vi "serial_AUCT_p4.vi"() -> ()   [LabVIEW 2018]
uses:
  Controls created/Control 3.ctl
  Controls created/Control 4.ctl
  <vilib>/Instr/_visa.llb/VISA Configure Serial Port (Instr).vi
  <instrlib>/LeCroy Wave Series/Public/Data/Read Single Waveform.vi
  <vilib>/Utility/file.llb/Write Delimited Spreadsheet (DBL).vi
  <instrlib>/Siglent SDG X Series/Siglent SDG X Series.lvlib
  <instrlib>/LeCroy Wave Series/LeCroy Wave Series.lvlib
panel:
  in  "Tab Control":enum32{"Page 1", "Page 2", "Page 3"}(tab)
  in  "VISA resource":refnum<visa-resource-name>="COM5"
  in  "NR":i16=10
  in  "Set Speed (Steps/s)":i16=900 min=0 max=3000 step=50
  in  "Baud Rate":u32=9600
  out "Iteration #":i32
  in  "NT":i16=10
  out "Error":errorcluster
  in  "Arbitray Movement":bool
  out "stop motion":bool
  in  "MOTION":bool
  in  "?":i8(slide) step=2 scale=0.0..2.0
  in  "OK Button":bool
  out "# NT":i32
  in  "Scanning Distance(in mm)":i32=26
  in  "ms to wait(Translation)":u32=100
  out "Dis_step":dbl
  in  "milliseconds to wait":u32=100
  in  "ms to wait(Rotation)":u32=100
  in  "Directory":string="E:\\Ankur\\Labview\\Automation\\Data"
  out "Code Part Time":dbl[](array[numeric])
  in  "VISA Refnum in":refnum<visa-resource-name>="USB0::0xF4EC::0xEE38::SDG2XCAD2R3765::INSTR"
  in  "Channel (1:Channel 1)":i32(ring)=1 items=["Channel 1"=1, "Channel 2"=2]
  in  "Enable Output (T: Enable)":bool=TRUE
  in  "Amplitude (1.0 Vpp)":dbl=20.0 format="%#.3f"
  in  "Frequency (1000 Hz)":T1=1500000.0 format="%#.6g"
  in  "DC Offset (0.00 V) in":dbl
  in  "Waveform Function (0: Sine) in":u16(ring) items=["Sine", "Square", "Ramp", "DC", "Pulse", "Arb"]
  in  "Phase (0.0 degrees)":dbl=0.002 min=-360.0 max=360.0 format="%#.1g"
  in  "Fall (20 ns)":dbl=8.4e-09 format="%#.3g"
  in  "Duty (20%)":dbl=4.32 min=0.0001 max=100.0 format="%.4g"
  in  "Delay (0.00 s)":dbl min=-1000000.0 max=1000000.0
  in  "Rise (20 ns)":dbl=1.04e-08 format="%#.3g"
  in  "True To \ngenerate\n pulse":T2=TRUE
  out "VISA resource name out":refnum<visa-resource-name>
  out "error out":errorcluster
  out "Output Filename":path
  out "error out 2":errorcluster
  in  "format string":string="Channel: %g \nWavetype: %g \nAMP: %gV\nFreq: %gHz \nRiseTime: %gs \nFallTime: %gs \nDutyCycle: %g"
  out "Output Directory":path
  in  "File Directory":path=path "E:/Ankur/Labview/Automation/Data/Exp1"
  in  "Filename 2":string="wave_data"
  out "Oscilloscope\n Runnning":bool
  in  "stop":bool
  out "Waveform Data":waveform(dbl)(graph)
  in  "Source (0: Channel 1)":u16(ring) items=["Channel 1", "Channel 2", "Channel 3", "Channel 4", "Memory 1", "Memory 2", "Memory 3", "Memory 4", "Function 1", "Function 2", "Function 3", "Function 4", "Function 5", "Function 6", "Function 7", "Function 8"]
  in  "Perform Auto Setup?":bool
  in  "Save Files in Directory (In Oscilloscope)":string="D:\\Automation\\Data"
  in  "Filename":string="Title"
  in  "Path to save DATA":path=path "E:/Ankur/Labview/Automation/Files/Oscdata"
  out "Saved filename":string
  in  "Save File locally":bool
  out "Error Dsocom":errorcluster
  in  "VISA resource name":refnum<visa-resource-name>="LecroyHDO4024-1"
  in  "Reset Scope?":bool
  out "VISA DSO":refnum<visa-resource-name>
  # "For Rotational motion"
  # "For Translational Motion"
  # "For Translational motion"
  # "OFF"
  # "ON"
  # "Instr conn"
  # "Scan. loop"
  # "All Comb"
  # "Yes"
  # "No"
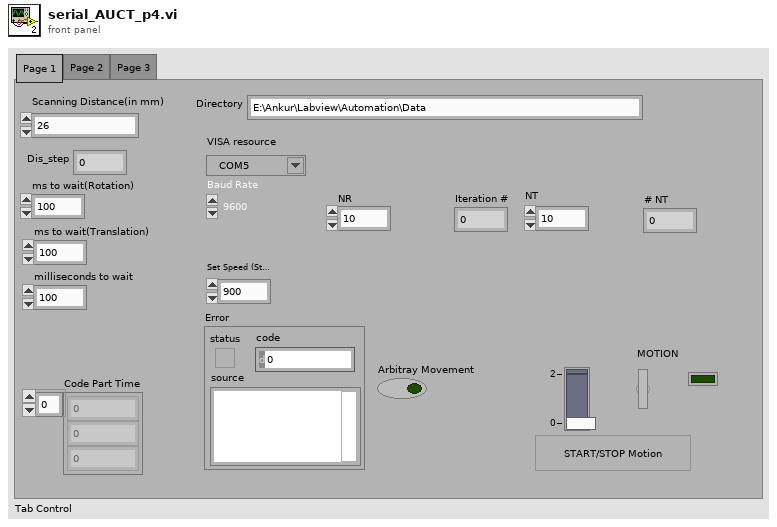
[diagram p1: front panel]
types:
  T1 = typedef "Control 3.ctl" = dbl
  T2 = typedef "Control 4.ctl" = bool
  T3 = enum16{"open", "replace", "create", "open or create", "replace or create", "replace or create with confirmation"}
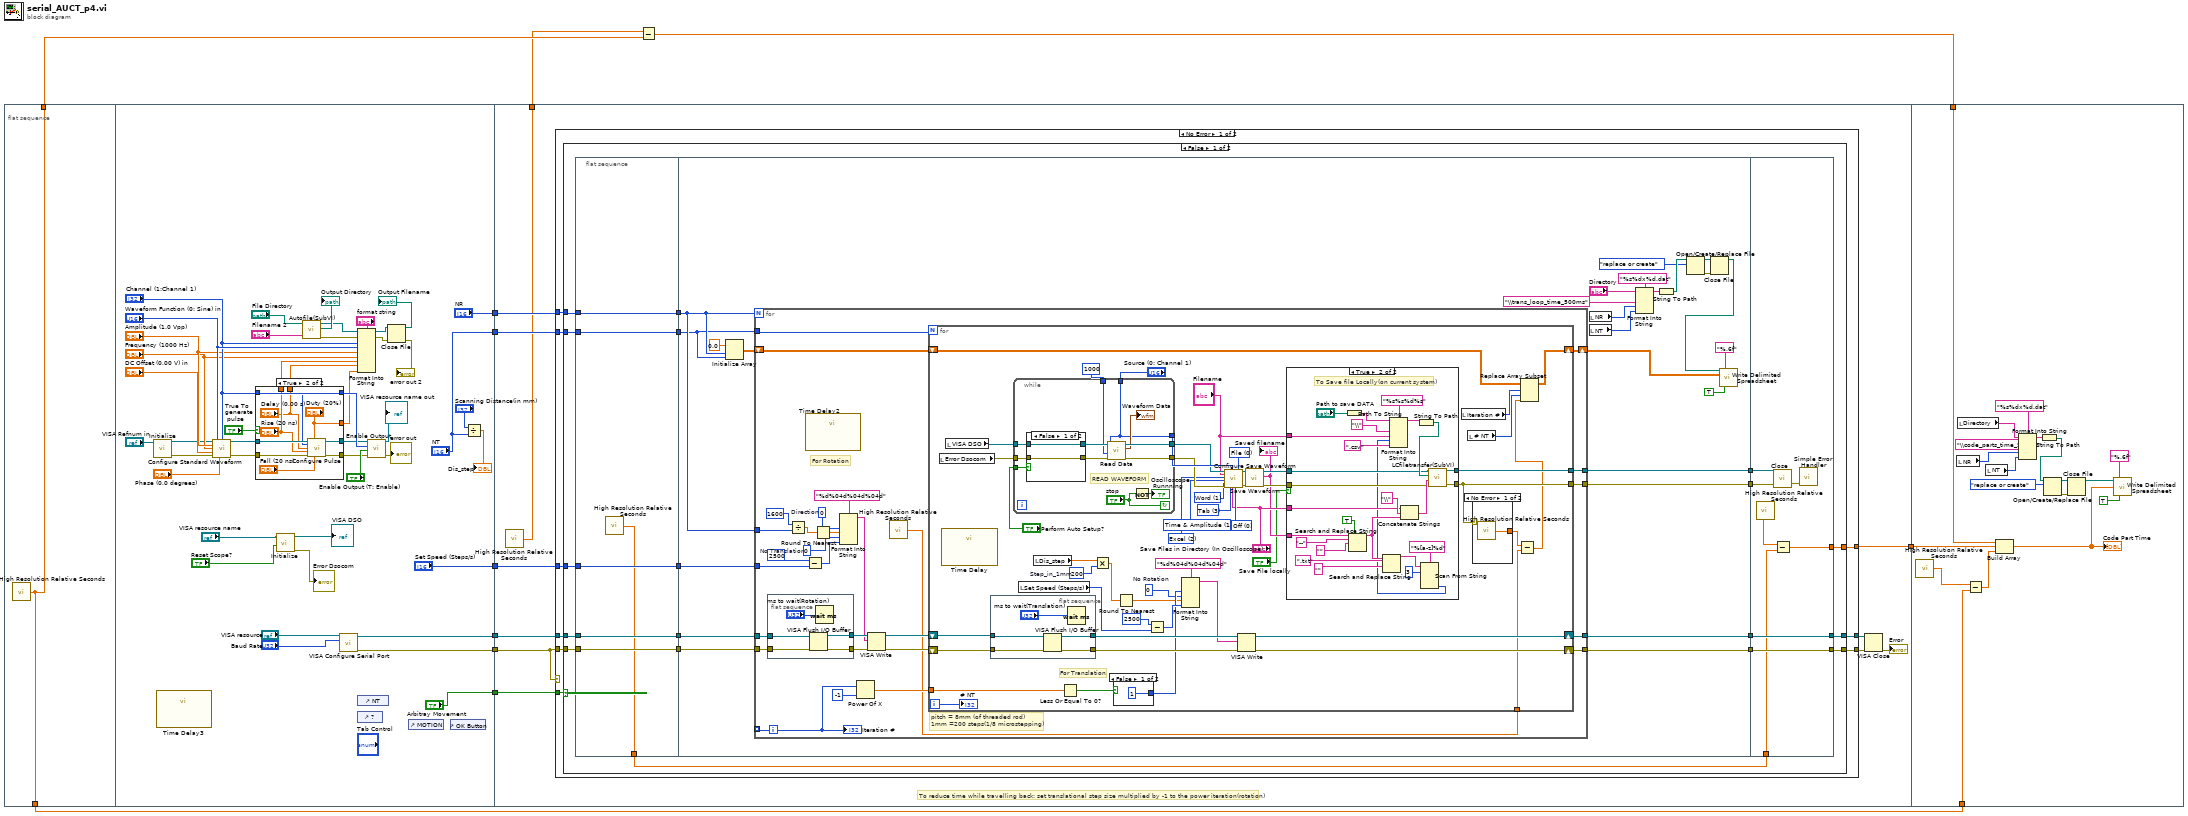
[diagram p0: block diagram]
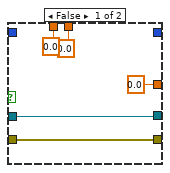
[diagram p2: hidden frame]
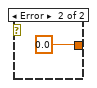
[diagram p3: hidden frame]
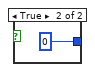
[diagram p4: hidden frame]
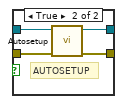
[diagram p6: hidden frame]
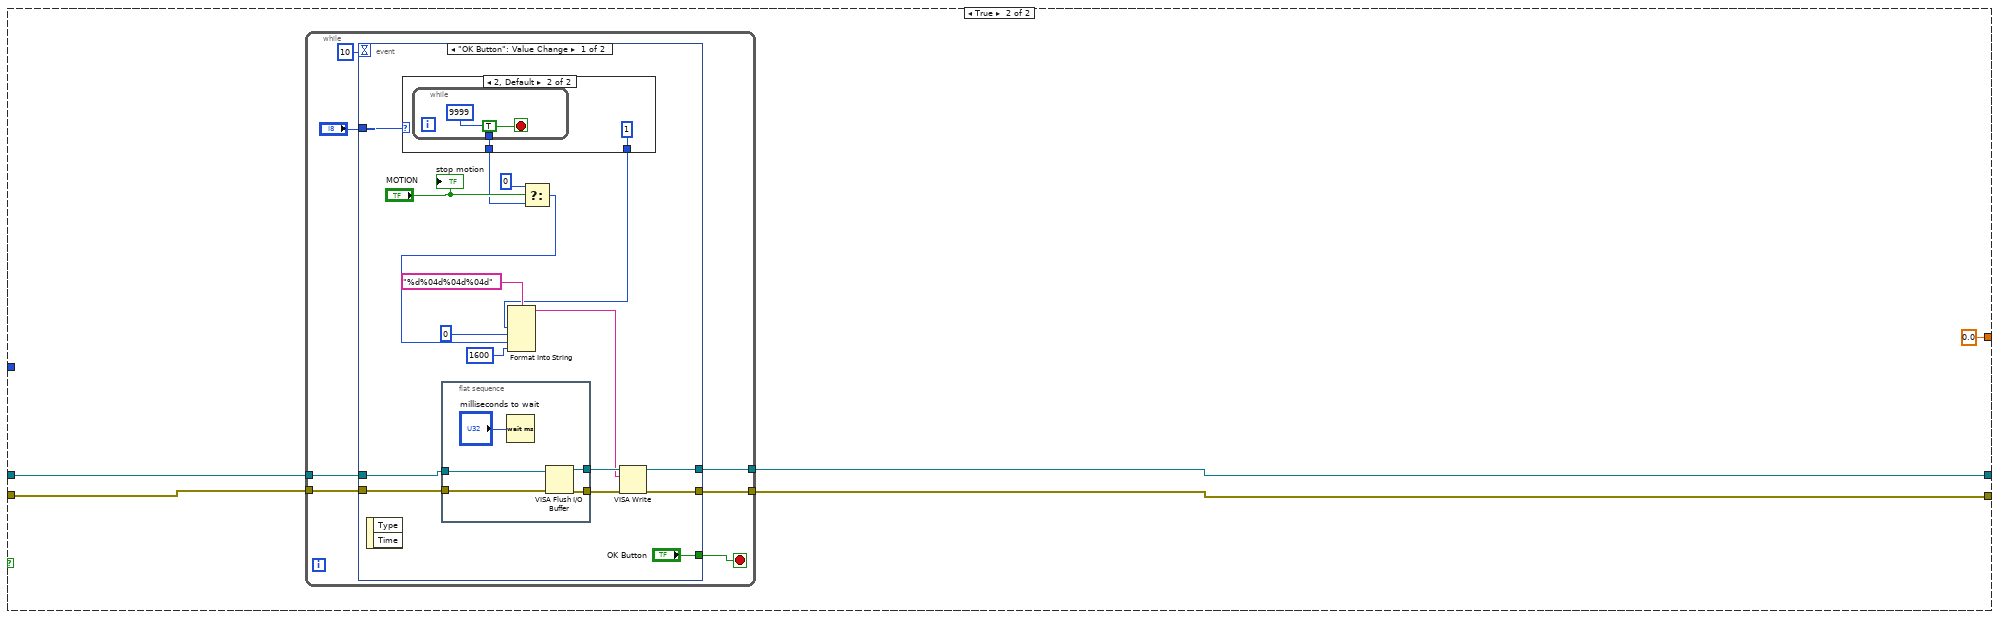
[diagram p7: hidden frame]
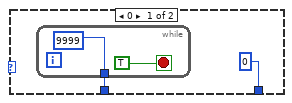
[diagram p8: hidden frame]
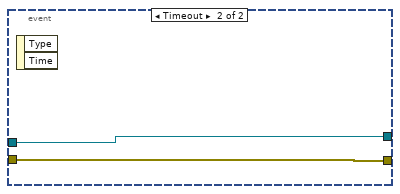
[diagram p9: hidden frame]
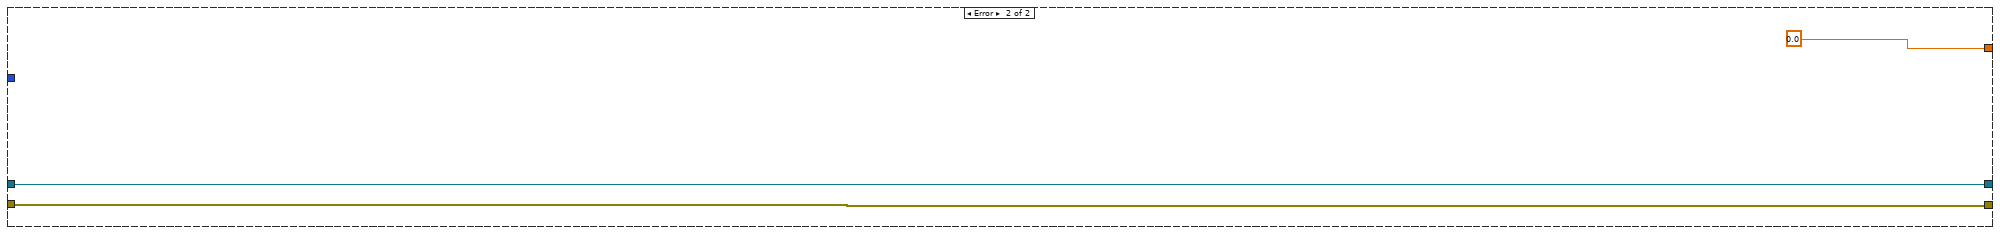
[diagram p10: hidden frame]
diagram:
  n1 = flat-sequence {
    tunnel: [w12] -> w3
    tunnel: [w12] -> w2
    tunnel: ["NT"] -> w11
    tunnel: [w17] -> w10
    tunnel: [w16] -> w9
    tunnel: ["Arbitray Movement"] -> w8
    tunnel: ["Set Speed (Steps/s)"] -> w7
    tunnel: ["NR"] -> w6
    tunnel: w11 -> [w78]
    tunnel: w10 -> [w77]
    tunnel: w9 -> [w76]
    tunnel: w8 -> [w75]
    tunnel: w7 -> [w74]
    tunnel: w6 -> [w73]
    tunnel: [w72] -> w4
    tunnel: [w71] -> w1
    tunnel: w5 -> [w351]
    tunnel: w4 -> [w350]
    tunnel: w3 -> [w349]
    frame #0 {
      n2 = call <vilib>:"High Resolution Relative Seconds.vi"() -> ("relative seconds"=w12:dbl)
    }
    frame #1 {
      n3 = call <instrlib>:"Initialize.vi"("VISA resource name"="VISA Refnum in") -> ("error out"=w24:errorcluster, "VISA resource name out"=w23:refnum<visa-resource-name>)  [unwired: 9 in]
      n4 = call "Time Delay3"() -> ()  [unwired: 11 in, 1 out]
      n5 = call <instrlib>:"Configure Standard Waveform.vi"("VISA resource name"=w23, "Waveform Function (0: Sine)"="Waveform Function (0: Sine) in", "Channel (1:Channel 1)"="Channel (1:Channel 1)", "Amplitude (1.0 Vpp)"="Amplitude (1.0 Vpp)", "Frequency (1000 Hz)"="Frequency (1000 Hz)", "DC Offset (0.00 V)"="DC Offset (0.00 V) in", "error in (no error)"=w24, "Phase (0.0 degrees)"="Phase (0.0 degrees)") -> ("VISA resource name out"=w28:refnum<visa-resource-name>, "error out"=w25:errorcluster)  [unwired: 6 in]
      n6 = case shown="True" "True To \ngenerate\n pulse" {
        tunnel: [w61 w69] -> w19
        tunnel: [w60 w68] -> w20
        tunnel: w28 -> [w61 w67]
        tunnel: w25 -> [w60 w66]
        tunnel: "Channel (1:Channel 1)" -> [_ w65]
        tunnel: "Channel (1:Channel 1)" -> [_ _]
        tunnel: [0.0 ("Duty (20%)") "Duty (20%)"] -> w32
        tunnel: [0.0 ("Rise (20 ns)") "Rise (20 ns)"] -> w40
        tunnel: [0.0 ("Delay (0.00 s)") "Delay (0.00 s)"] -> w41
        frame False {
        }
        frame True {
          n7 = call <instrlib>:"Configure Pulse.vi"("VISA resource name"=w67, "Duty (20%)"="Duty (20%)", "Channel (1:Channel 1)"=w65, "Delay (0.00 s)"="Delay (0.00 s)", "Rise (20 ns)"="Rise (20 ns)", "error in (no error)"=w66, "Fall (20 ns)"="Fall (20 ns)") -> ("VISA resource name out"=w69:refnum<visa-resource-name>, "error out"=w68:errorcluster)  [unwired: 7 in]
        }
      }
      n8 = call <instrlib>:"Initialize.vi"("Reset? (T: Yes)"="Reset Scope?", "VISA resource name"="VISA resource name") -> ("error out"=→"Error Dsocom":errorcluster, "VISA resource name out"=→"VISA DSO":refnum<visa-resource-name>)  [unwired: 8 in]
      n9 = call "Autofile(SubVI).vi"("Filename"="Filename 2", "File Directory"="File Directory") -> ("error out"=w45:errorcluster, "Output Directory"=→"Output Directory":path, "Byte Stream File out"=w44:refnum<file>)  [unwired: 7 in]
      n10 = call-poly "VISA Configure Serial Port"("VISA resource name"="VISA resource", "baud rate (9600)"="Baud Rate") -> ("VISA resource name out"=w17:refnum<visa-resource-name>, "error out"=w16:errorcluster)  [unwired: 12 in]
      n11 = Format Into String(format string="format string", initial string=w44, error in=w45, "Channel (1:Channel 1)", "Waveform Function (0: Sine) in", "Amplitude (1.0 Vpp)", "Frequency (1000 Hz)", w40, w41, w32) -> (resulting string=w33:refnum<file>, error out=w36:errorcluster)
      n12 = control-ref of="NT"() -> ()  [unwired: 1 out]
      n13 = control-ref of="?"() -> ()  [unwired: 1 out]
      n14 = call <instrlib>:"Enable Output.vi"("error in (no error)"=w20, "Enable Output (T: Enable)"="Enable Output (T: Enable)", "Channel (1:Channel 1)"="Channel (1:Channel 1)", "VISA resource name"=w19) -> ("error out"=→"error out":errorcluster, "VISA resource name out"=→"VISA resource name out":refnum<visa-resource-name>)  [unwired: 6 in]
      n15 = Close File(refnum=w33, error in=w36) -> (path=→"Output Filename":path, error out=→"error out 2":errorcluster)
      n16 = control-ref of="MOTION"() -> ()  [unwired: 1 out]
      n17 = control-ref of="OK Button"() -> ()  [unwired: 1 out]
      n18 = Divide(x="Scanning Distance(in mm)", y="NT") -> (x/y=→"Dis_step":dbl)
    }
    frame #2 {
      # "To reduce time while travelling back: set translational step size multiplied by -1 to the power iteration(rotation)"
      n19 = call <vilib>:"High Resolution Relative Seconds.vi"() -> ("relative seconds"=w71:dbl)
      n20 = case shown="No Error" w76 {
        tunnel: [w83 w333] -> w81
        tunnel: w73 -> [w90 _]
        tunnel: w74 -> [w89 _]
        tunnel: w75 -> [w88 _]
        tunnel: w76 -> [w87 w333]
        tunnel: w77 -> [w86 w332]
        tunnel: w78 -> [w85 _]
        tunnel: [w84 w332] -> w79
        tunnel: [w82 0.0] -> w72
        frame No Error {
          n21 = case shown="False" w88 {
            tunnel: w90 -> [w105 _]
            tunnel: w89 -> [w108 _]
            tunnel: w87 -> [w107 w291]
            tunnel: w86 -> [w106 w290]
            tunnel: w85 -> [w104 _]
            tunnel: [w103 w289] -> w84
            tunnel: [w93 w288] -> w83
            tunnel: [w92 0.0] -> w82
            frame False {
              n22 = flat-sequence {
                tunnel: w104 -> [w110]
                tunnel: w105 -> [w111]
                tunnel: w106 -> [w112]
                tunnel: w107 -> [w113]
                tunnel: w108 -> [w114]
                tunnel: [w114] -> w100
                tunnel: [w113] -> w99
                tunnel: [w112] -> w98
                tunnel: [w111] -> w97
                tunnel: [w110] -> w96
                tunnel: [w109] -> w91
                tunnel: [w136] -> w102
                tunnel: [w135] -> w101
                tunnel: w100 -> [w139]
                tunnel: w99 -> [w138]
                tunnel: w98 -> [w137]
                tunnel: w97 -> [w132]
                tunnel: w96 -> [w130]
                tunnel: [w134] -> w95
                tunnel: [w133] -> w94
                tunnel: [w286] -> w103
                tunnel: w102 -> [w286]
                tunnel: w101 -> [w282]
                tunnel: w95 -> [w284]
                tunnel: w94 -> [w283]
                tunnel: [w282] -> w93
                tunnel: [w280] -> w92
                tunnel: w91 -> [w279]
                frame #0 {
                  n23 = call <vilib>:"High Resolution Relative Seconds.vi"() -> ("relative seconds"=w109:dbl)
                }
                frame #1 {
                  n24 = Initialize Array(0.0, w132, w130) -> (w116:dbl[][])
                  n25 = for {
                    N: w132 -> [_]
                    tunnel: [w164] -> w135
                    tunnel: [w165] -> w136
                    tunnel: w139 -> [w145]
                    tunnel: [w167] -> _ mode=indexing
                    tunnel: w138 -> [w158]
                    tunnel: w137 -> [w159]
                    tunnel: w132 -> [w151]
                    tunnel: w130 -> [w147]
                    tunnel: [w144] -> w134
                    tunnel: [w143] -> w133
                    shift-right: [w140] -> w115
                    shift-left: w116 -> [w141]
                    i -> [w167]
                    w155 = 0  # No Translation
                    w153 = 0  # Direction
                    # "pitch = 8mm (of threaded rod)\n1mm =200 steps(1/8 microstepping)"
                    # "For Rotation"
                    n26 = flat-sequence {
                      tunnel: [w172] -> w162
                      tunnel: [w171] -> w163
                      tunnel: w159 -> [w169]
                      tunnel: w158 -> [w168]
                      frame #0 {
                        n27 = VISA Flush I/O Buffer(VISA resource name=w169, error in (no error)=w168) -> (VISA resource name out=w172:refnum<visa-resource-name>, error out=w171:errorcluster)  [unwired: 1 in]
                        n28 = Wait (ms)(milliseconds to wait="ms to wait(Rotation)") -> ()  [unwired: 1 out]
                      }
                    }
                    n29 = Divide(x=i16 1600, y=w151) -> (x/y=w150:dbl)
                    n30 = call "Time Delay2"() -> ()  [unwired: 11 in, 1 out]
                    n31 = Subtract(x=i16 2500 ("y"), y=w145) -> (x-y=w154:i16)
                    n32 = Round To Nearest(number=w150) -> (nearest integer value=w149:dbl)
                    n33 = Format Into String(format string="%d%04d%04d%04d", w153, w149, w155, w154) -> (resulting string=w157:string)  [unwired: 2 in, 1 out]
                    n34 = Power Of X(1:-1 ("x"), 2:w167) -> (0:w148:dbl)
                    n35 = VISA Write(VISA resource name=w162, write buffer=w157, error in (no error)=w163) -> (VISA resource name out=w160:refnum<visa-resource-name>, error out=w161:errorcluster)  [unwired: 1 out]
                    n36 = call <vilib>:"High Resolution Relative Seconds.vi"() -> ("relative seconds"=w142:dbl)
                    n37 = for {
                      N: w147 -> [_]
                      shift-right: [w192] -> w165
                      shift-left: w160 -> [w202]
                      shift-right: [w191] -> w164
                      shift-left: w161 -> [w201]
                      tunnel: w148 -> [w195]
                      tunnel: [w180] -> w144
                      tunnel: [w181] -> w143
                      tunnel: w142 -> [w178]
                      shift-right: [w176] -> w140
                      shift-left: w141 -> [w173]
                      i -> [w223]
                      w187 = 200  # Step_in_1mm
                      w190 = 0  # No Rotation
                      w213 = u16 3 items=["Comma", "Space", "Semicolon", "Tab"] ("Delimiter (  0:Comma)")
                      w212 = u16 0 items=["Off", "Wrap", "Fill"] ("Auto Save (0:Off")
                      w214 = u16 1 items=["Byte", "Word", "Auto"] ("BinarySubFormat (1: Word)")
                      w215 = u16 1 items=["Amplitude Only", "Time & Amplitude", "With Header"] ("SubFormat (1: Time & Amplitude)")
                      w216 = u16 2 items=["Binary", "ASCII", "Excel", "MATLAB", "MathCad", "WaveML"] ("Format (0: Binary)")
                      w211 = u16 0 items=["File", "M1", "M2", "M3", "M4"] ("Destination (0:File)")
                      # "For Translation"
                      n38 = local read "Error Dsocom"() -> (w182:errorcluster)
                      n39 = call "Time Delay"() -> ()  [unwired: 11 in, 1 out]
                      n40 = local read "VISA DSO"() -> (w183:refnum<visa-resource-name>)
                      n41 = flat-sequence {
                        tunnel: [w232] -> w200
                        tunnel: [w231] -> w199
                        tunnel: w202 -> [w229]
                        tunnel: w201 -> [w228]
                        frame #0 {
                          n42 = VISA Flush I/O Buffer(VISA resource name=w229, error in (no error)=w228) -> (VISA resource name out=w232:refnum<visa-resource-name>, error out=w231:errorcluster)  [unwired: 1 in]
                          n43 = Wait (ms)(milliseconds to wait="ms to wait(Translation)") -> ()  [unwired: 1 out]
                        }
                      }
                      n44 = while {
                        tunnel: [w270] -> w221
                        tunnel: [w269] -> w220
                        tunnel: "Perform Auto Setup?" -> [w268]
                        tunnel: "Source (0: Channel 1)" -> [w262]
                        tunnel: w183 -> [w267]
                        tunnel: u32 1000 ("Timeout (10000 ms)") -> [w266]
                        tunnel: [w262] -> w222
                        tunnel: w182 -> [w261]
                        stop <- "stop" continue-if-true
                        # "READ WAVEFORM"
                        n45 = case shown="False" w268 {
                          tunnel: w261 -> [w273 w278]
                          tunnel: w267 -> [w274 w277]
                          tunnel: [w274 w276] -> w272
                          tunnel: [w273 w275] -> w271
                          frame False {
                          }
                          frame True {
                            # "AUTOSETUP"
                            n46 = call <instrlib>:"Autosetup.vi"("error in (no error)"=w278, "VISA resource name"=w277) -> ("error out"=w275:errorcluster, "VISA resource name out"=w276:refnum<visa-resource-name>)  [unwired: 8 in]
                          }
                        }
                        n47 = call-poly <instrlib>:"Read Data.vi"("error in (no error)"=w271, "Timeout (10000 ms)"=w266, "Source (0: Channel 1)"=w262, "VISA resource name"=w272) -> ("error out"=w270:errorcluster, "Waveform Data"=→"Waveform Data":waveform(dbl), "VISA resource name out"=w269:refnum<visa-resource-name>)  [unwired: 5 in]
                        n48 = Not(x="stop") -> (.not. x?=→"Oscilloscope\n Runnning":bool)
                      }
                      n49 = local read "Set Speed (Steps/s)"() -> (w184:i16)
                      n50 = local read "Dis_step"() -> (w188:dbl)
                      n51 = Less Or Equal To 0?(x=w195) -> (x <= 0?=w194:bool)
                      n52 = Multiply(x=w188, y=w187) -> (x*y=w186:dbl)
                      n53 = case shown="False" w194 {
                        tunnel: [1 0] -> w193
                        frame False {
                        }
                        frame True {
                        }
                      }
                      n54 = Round To Nearest(number=w186) -> (nearest integer value=w189:dbl)
                      n55 = Subtract(x=i16 2500 ("y"), y=w184) -> (x-y=w198:i16)
                      n56 = Format Into String(format string="%d%04d%04d%04d", w193, w190, w189, w198) -> (resulting string=w196:string)  [unwired: 2 in, 1 out]
                      n57 = call <instrlib>:"Configure Save Waveform.vi"("VISA resource name"=w220, "Trace Title (Title)"="Filename", "Format (0: Binary)"=w216, "SubFormat (1: Time & Amplitude)"=w215, "BinarySubFormat (1: Word)"=w214, "error in (no error)"=w221, "Delimiter (  0:Comma)"=w213, "Source (0: Channel 1)"=w222, "Save Files in Directory (D:\\Waveforms)"="Save Files in Directory (In Oscilloscope)", "Auto Save (0:Off"=w212, "Destination (0:File)"=w211) -> ("VISA resource name out"=w210:refnum<visa-resource-name>, "error out"=w209:errorcluster)  [unwired: 7 in]
                      n58 = VISA Write(VISA resource name=w200, write buffer=w196, error in (no error)=w199) -> (VISA resource name out=w192:refnum<visa-resource-name>, error out=w191:errorcluster)  [unwired: 1 out]
                      n59 = call <instrlib>:"Save Waveform.vi"("error in (no error)"=w209, "VISA resource name"=w210) -> ("error out"=w207:errorcluster, "Saved filename"=w205:string, "VISA resource name out"=w206:refnum<visa-resource-name>)  [unwired: 7 in]
                      "Saved filename" <- w205
                      n60 = case shown="True" "Save File locally" {
                        tunnel: [w234 w257] -> w181
                        tunnel: [w233 w256] -> w180
                        tunnel: "Save Files in Directory (In Oscilloscope)" -> [_ w250]
                        tunnel: w207 -> [w233 w249]
                        tunnel: w206 -> [w234 w248]
                        tunnel: w205 -> [_ w247]
                        tunnel: "Filename" -> [_ w246]
                        frame False {
                        }
                        frame True {
                          # "To Save file Locally(on current system)"
                          n61 = Path To String(path="Path to save DATA") -> (string=w251:string)
                          n62 = Search and Replace String(replace all?=TRUE ("replace all? (F)"), input string=w247, search string="--", replace string="" ("replace string (\"\")")) -> (result string=w242:string)  [unwired: 4 in, 3 out]
                          n63 = Search and Replace String(input string=w242, search string=".txt", replace string="" ("replace string (\"\")")) -> (result string=w245:string)  [unwired: 5 in, 3 out]
                          n64 = Concatenate Strings(w250, "\\" ("string"), w242) -> (w258:string)
                          n65 = Scan From String(format string="%[a-z]%d", input string=w245, initial scan location=u32 3) -> (output 2=w238:i32)  [unwired: 4 in, 3 out]
                          n66 = Format Into String(format string="%s%s%d%s", initial string=w251, "\\" ("input 1"), w246, w238, ".csv" ("input 3")) -> (resulting string=w237:string)  [unwired: 1 in, 1 out]
                          n67 = String To Path(string=w237) -> (path=w255:path)
                          n68 = call <userlib>:"LCfiletransfer(SubVI).vi"("error in (no error)"=w249, "Source Filename"=w258, "file path (use dialog)"=w255, "VISA Refnum in"=w248) -> ("error out"=w256:errorcluster, "VISA Refnum out"=w257:refnum<visa-resource-name>)  [unwired: 5 in, 1 out]
                        }
                      }
                      n69 = local read "Iteration #"() -> (w177:i32)
                      n70 = local read "# NT"() -> (w175:i32)
                      n71 = case shown="No Error" w180 {
                        tunnel: [w224 0.0] -> w179
                        frame No Error {
                          n72 = call <vilib>:"High Resolution Relative Seconds.vi"() -> ("relative seconds"=w224:dbl)
                        }
                        frame Error {
                        }
                      }
                      n73 = Subtract(x=w179, y=w178) -> (x-y=w174:dbl)
                      n74 = Replace Array Subset(array=w173, new element=w174, index (row)=w177, index (col)=w175) -> (w176:dbl[][])
                      "# NT" <- w223
                    }
                    "Iteration #" <- w167
                  }
                  n75 = local read "NR"() -> (w125:i16)
                  n76 = local read "NT"() -> (w126:i16)
                  n77 = Format Into String(format string="%s%dx%d.dat", initial string="Directory", "\\trans_loop_time_500ms", w125, w126) -> (resulting string=w128:string)  [unwired: 1 in, 1 out]
                  n78 = String To Path(string=w128) -> (path=w129:path)
                  n79 = Open/Create/Replace File(file path (use dialog)=w129, operation (0:open)=T3."replace or create") -> (refnum out=w120:refnum<file>, error out=w121:errorcluster)  [unwired: 4 in, 1 out]
                  n80 = Close File(refnum=w120, error in=w121) -> (path=w119:path)  [unwired: 1 out]
                  n81 = call-poly <vilib>:"Write Delimited Spreadsheet.vi"("file path (dialog if empty)"=w119, "format (%.3f)"="%.6f", "2D data"=w115, "transpose? (no:F)"=TRUE) -> ()  [unwired: 10 in, 2 out]
                }
                frame #2 {
                  n82 = call <vilib>:"High Resolution Relative Seconds.vi"() -> ("relative seconds"=w281:dbl)
                  n83 = call <instrlib>:"Close.vi"("error in (no error)"=w284, "VISA resource name"=w283) -> ("error out"=w285:errorcluster)  [unwired: 9 in]
                  n84 = Subtract(x=w281, y=w279) -> (x-y=w280:dbl)
                  n85 = call <vilib>:"Simple Error Handler.vi"("error in (no error)"=w285) -> ()  [unwired: 4 in, 5 out]
                }
              }
            }
            frame True {
              n86 = while {
                tunnel: w291 -> [w296]
                tunnel: w290 -> [w295]
                tunnel: [w293] -> w289
                tunnel: [w294] -> w288
                stop <- w292 stop-if-true
                n87 = event shown="[0] \"OK Button\": Value Change" {
                  selector: _ -> [_ _]
                  dyn-events: _ -> [_ _]
                  timeout: 10 -> [_ _]
                  tunnel: "?" -> [w314 _]
                  tunnel: w296 -> [w304 w329]
                  tunnel: w295 -> [w305 w330]
                  tunnel: [w302 w329] -> w294
                  tunnel: [w303 w330] -> w293
                  tunnel: ["OK Button" _] -> w292
                  event "OK Button": Value Change {
                    n88 = event-data() -> ()  [unwired: 1 in, 2 out]
                    n89 = case shown="2, Default" w314 {
                      tunnel: [w322 w326] -> w312
                      tunnel: [0 ("input 1") 1 ("input 1")] -> w300
                      frame 0 {
                        n90 = while {
                          tunnel: [i16 9999 ("# of Steps to Move")] -> w322
                          stop <- TRUE ("Stop Reverse movement") stop-if-true
                        }
                      }
                      frame 2, Default {
                        n91 = while {
                          tunnel: [i16 9999 ("# of Steps to Move")] -> w326
                          stop <- TRUE ("Stop Forward movement") stop-if-true
                        }
                      }
                    }
                    n92 = flat-sequence {
                      tunnel: [w320] -> w311
                      tunnel: [w319] -> w310
                      tunnel: w305 -> [w317]
                      tunnel: w304 -> [w316]
                      frame #0 {
                        n93 = Wait (ms)(milliseconds to wait="milliseconds to wait") -> ()  [unwired: 1 out]
                        n94 = VISA Flush I/O Buffer(VISA resource name=w317, error in (no error)=w316) -> (VISA resource name out=w320:refnum<visa-resource-name>, error out=w319:errorcluster)  [unwired: 1 in]
                      }
                    }
                    n95 = Select(t=0, s="MOTION", f=w312) -> (s? t:f=w301:i32)
                    n96 = Format Into String(format string="%d%04d%04d%04d", w300, 0 ("input 2"), w301, 1600 ("input 4")) -> (resulting string=w308:string)  [unwired: 2 in, 1 out]
                    n97 = VISA Write(VISA resource name=w311, write buffer=w308, error in (no error)=w310) -> (VISA resource name out=w303:refnum<visa-resource-name>, error out=w302:errorcluster)  [unwired: 1 out]
                    "stop motion" <- "MOTION"
                  }
                  event Timeout {
                    n98 = event-data() -> ()  [unwired: 1 in, 2 out]
                  }
                }
              }
            }
          }
        }
        frame Error {
        }
      }
      n99 = VISA Close(VISA resource name=w79, error in (no error)=w81) -> (error out=→"Error":errorcluster)
    }
    frame #3 {
      n100 = call <vilib>:"High Resolution Relative Seconds.vi"() -> ("relative seconds"=w348:dbl)
      n101 = local read "NR"() -> (w337:i16)
      n102 = local read "Directory"() -> (w334:string)
      n103 = Subtract(x=w348, y=w349) -> (x-y=w352:dbl)
      n104 = local read "NT"() -> (w336:i16)
      n105 = Build Array(w351, w350, w352) -> (w338:dbl[])
      "Code Part Time" <- w338
      n106 = Format Into String(format string="%s%dx%d.dat", initial string=w334, "\\code_parts_time_500ms", w337, w336) -> (resulting string=w340:string)  [unwired: 1 in, 1 out]
      n107 = String To Path(string=w340) -> (path=w339:path)
      n108 = Open/Create/Replace File(file path (use dialog)=w339, operation (0:open)=T3."replace or create") -> (refnum out=w346:refnum<file>, error out=w347:errorcluster)  [unwired: 4 in, 1 out]
      n109 = Close File(refnum=w346, error in=w347) -> (path=w343:path)  [unwired: 1 out]
      n110 = call-poly <vilib>:"Write Delimited Spreadsheet.vi"("file path (dialog if empty)"=w343, "format (%.3f)"="%.6f", "1D data"=w338, "transpose? (no:F)"=TRUE) -> ()  [unwired: 10 in, 2 out]
    }
  }
  n111 = Subtract(x=w1, y=w2) -> (x-y=w5:dbl)
